vi "Polling Core.vi"(8 "Error In":errorcluster, 11 "BNT_ULx-MCSV-Ctr2Freq in":refnum<class "BNT_ULx-MCSV-Ctr2Freq.lvclass">) -> (0 "Error Out":errorcluster, 3 "BNT_ULx-MCSV-Ctr2Freq in":refnum<class "BNT_ULx-MCSV-Ctr2Freq.lvclass">)   [LabVIEW 2020, in "BNT_ULx.lvlib" / "BNT_ULx-MCSV-Ctr2Freq.lvclass"]
uses:
  BNT_ULx-MCSV-Ctr2Freq.lvclass
  BNT_ULx-MCSV-Ctr2Freq.lvclass/BNT_ULx-MCSV-Ctr2Freq.ctl
  CSPP_Core/Classes/CSPP_ProcessVariables/PVConnection/PVConnection.lvclass
  CSPP_Core/Classes/CSPP_ProcessVariables/ProcessVariable/PV.lvclass
  BNT_ULx-MCSV/BNT_ULx-MCSV.lvclass
  C:/User/Brand/LVP/CSPP/CSPP-Template/Packages/BNT_ULx/BNT_ULx-MCSV/BNT_ULx-MCSV/BNT_ULx-MCSV.lvclass
  C:/User/Brand/LVP/CSPP/CSPP-Template/Packages/CSPP_Core/Actors/CSPP_DeviceActor/CSPP_DeviceActor.lvclass
  C:/User/Brand/LVP/CSPP/CSPP-Template/Packages/CSPP_Core/Actors/CSPP_BaseActor/CSPP_BaseActor.lvclass
  C:/Program Files (x86)/National Instruments/LabVIEW 2020/vi.lib/ActorFramework/Actor/Actor.lvclass
  C:/User/Brand/LVP/CSPP/CSPP-Template/Packages/BNT_ULx/BNT_ULx-MCSV/BNT_ULx-MCSV-Ctr2Freq/BNT_ULx-MCSV-Ctr2Freq.lvclass
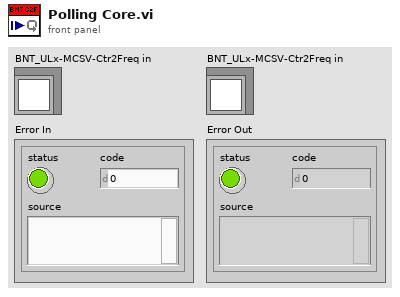
[diagram p1: front panel]
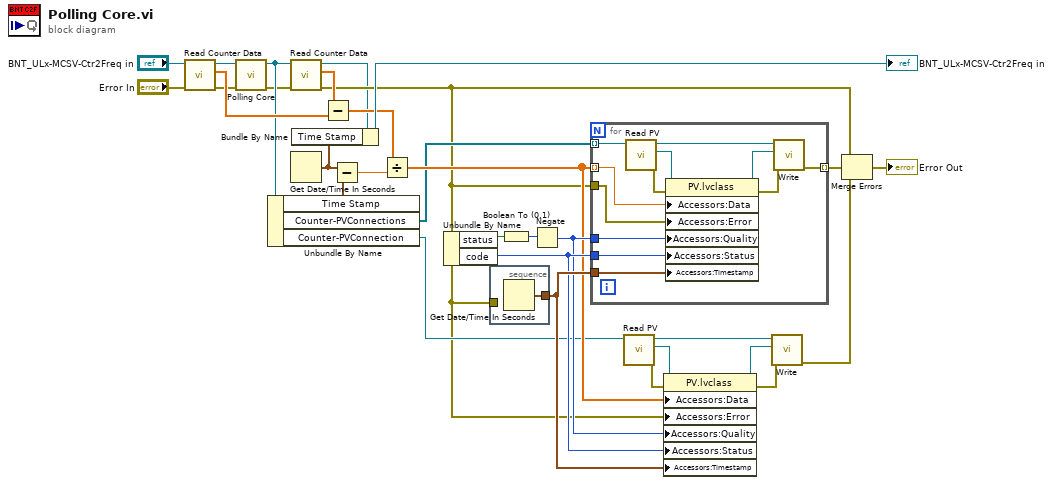
[diagram p0: block diagram]
diagram:
  n1 = call "Read Counter Data.vi"("error in (no error)"="Error In", "BNT_DAQmx-MCSV in"="BNT_ULx-MCSV-Ctr2Freq in") -> ("error out"=w6:errorcluster, "Counter Data"=w9:dbl[], "BNT_DAQmx-MCSV out"=w8:refnum<class "BNT_ULx-MCSV-Ctr2Freq.lvclass">)  [unwired: 7 in]
  n2 = call-parent "Polling Core.vi"("Error In"=w6, "BNT_DAQmx-MCSV in"=w8) -> ("Error Out"=w3:errorcluster, "BNT_DAQmx-MCSV out"=w4:refnum<class "BNT_ULx-MCSV-Ctr2Freq.lvclass">)  [unwired: 8 in]
  n3 = Unbundle By Name(w4) -> ("Time Stamp"=w31:timestamp, "Counter-PVConnections"=w16:refnum<class "PVConnection.lvclass">[], "Counter-PVConnection"=w15:refnum<class "PVConnection.lvclass">)
  n4 = call "Read Counter Data.vi"("error in (no error)"=w3, "BNT_DAQmx-MCSV in"=w4) -> ("error out"=w2:errorcluster, "Counter Data"=w5:dbl[], "BNT_DAQmx-MCSV out"=w1:refnum<class "BNT_ULx-MCSV-Ctr2Freq.lvclass">)  [unwired: 7 in]
  n5 = Get Date/Time In Seconds() -> (seconds since 1Jan1904=w14:timestamp)
  n6 = Bundle By Name(cluster=w1, "Time Stamp"=w14) -> (→"BNT_ULx-MCSV-Ctr2Freq in":refnum<class "BNT_ULx-MCSV-Ctr2Freq.lvclass">)
  n7 = Subtract(x=w5, y=w9) -> (x-y=w11:dbl[])
  n8 = Subtract(x=w14, y=w31) -> (x-y=w30:dbl)
  n9 = Divide(x=w11, y=w30) -> (x/y=w17:dbl[])
  n10 = Unbundle By Name(w2) -> ("status"=w19:bool, "code"=w27:i32)
  n11 = stacked-sequence {
    tunnel: [w32] -> w28
    tunnel: w2 -> [_]
    frame #0 {
      n12 = Get Date/Time In Seconds() -> (seconds since 1Jan1904=w32:timestamp)
    }
  }
  n13 = Boolean To (0,1)(Boolean=w19) -> (0, 1=w18:i16)
  n14 = Negate(x=w18) -> (-x=w26:i16)
  n15 = for {
    tunnel: w16 -> [w36] mode=indexing
    tunnel: w17 -> [w44] mode=indexing
    tunnel: w2 -> [w43]
    tunnel: [w40] -> w20 mode=indexing
    tunnel: w26 -> [w39]
    tunnel: w27 -> [w38]
    tunnel: w28 -> [w37]
    n16 = call "Read PV.vi"("PVConnection in"=w36) -> ("error out"=w33:errorcluster, "PV"=w34:refnum<class "PV.lvclass">, "PVConnection out"=w35:refnum<class "PVConnection.lvclass">)  [unwired: 8 in]
    n17 = property class="PV.lvclass"(reference=w34, error in=w33, "Accessors:Data"=w44, "Accessors:Error"=w43, "Accessors:Quality"=w39, "Accessors:Status"=w38, "Accessors:Timestamp"=w37) -> (reference out=w42:refnum<class "PV.lvclass">, error out=w41:errorcluster)
    n18 = call "Write.vi"("error in (no error)"=w41, "PV"=w42, "PVConnection in"=w35) -> ("error out"=w40:errorcluster)  [unwired: 6 in, 2 out]
  }
  n19 = call "Read PV.vi"("PVConnection in"=w15) -> ("error out"=w21:errorcluster, "PV"=w22:refnum<class "PV.lvclass">, "PVConnection out"=w23:refnum<class "PVConnection.lvclass">)  [unwired: 8 in]
  n20 = property class="PV.lvclass"(reference=w22, error in=w21, "Accessors:Data"=w17, "Accessors:Error"=w2, "Accessors:Quality"=w26, "Accessors:Status"=w27, "Accessors:Timestamp"=w28) -> (reference out=w25:refnum<class "PV.lvclass">, error out=w24:errorcluster)
  n21 = call "Write.vi"("error in (no error)"=w24, "PV"=w25, "PVConnection in"=w23) -> ("error out"=w29:errorcluster)  [unwired: 6 in, 2 out]
  n22 = Merge Errors(w2, w20, w29) -> (→"Error Out":errorcluster)
